vi "FL_Decode_RAW_to_DEC_2.vi"(0 "SB size (loc. var. only)":u8, 1 "IO ports config":bool[](array[boolean])=[TRUE, TRUE, FALSE, FALSE], 2 "Input string":string, 3 "Input timestamp":timestamp, 4 "IO inversion config.":u16, 5 "Error In":errorcluster) -> (6 "Output string leftover":string, 7 "DEC output cluster":T1, 8 "Error Out":errorcluster)   [LabVIEW 2018, in "Tracker.lvlib"]
uses:
  Tracker.lvlib
  Controls/CTL_Decoded_data_frame.ctl
panel:
  out "TTL ins":bool[](array[boolean])
  out "TTL outs":bool[](array[boolean])
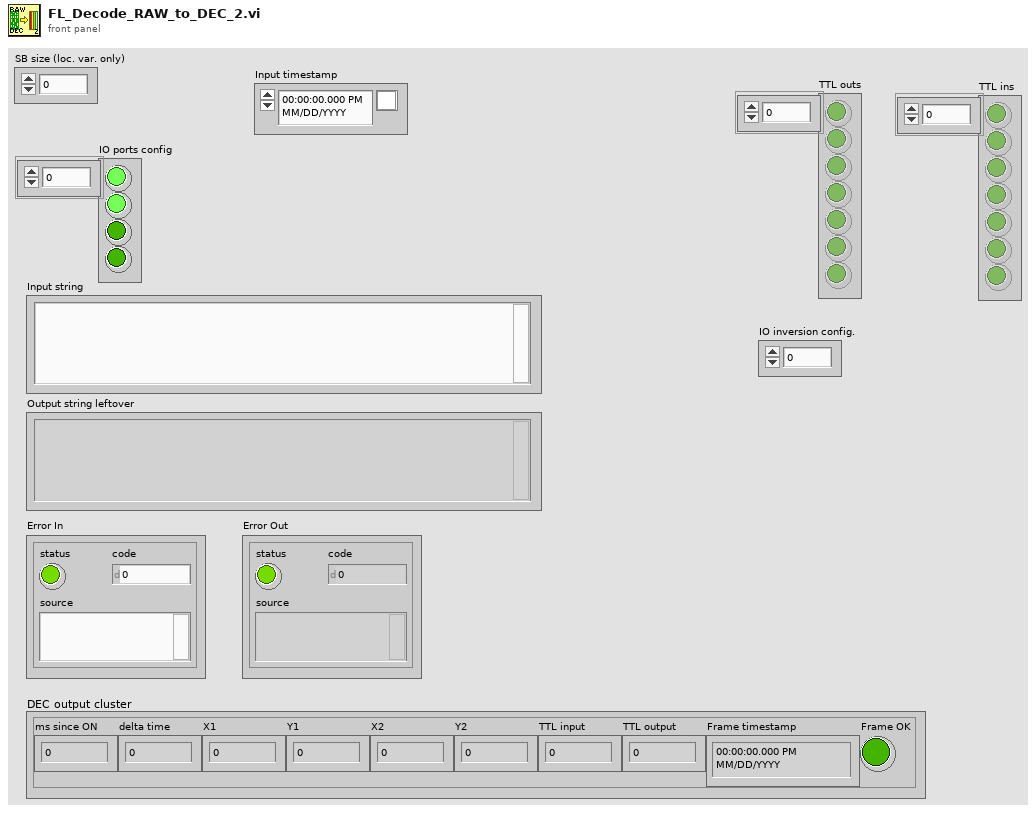
[diagram p1: front panel]
types:
  T1 = typedef "Tracker.lvlib/CTL_Decoded_data_frame.ctl" = cluster{"ms since ON":u32, "delta time":u32, "X1":sgl, "Y1":sgl, "X2":sgl, "Y2":sgl, "TTL input":i16, "TTL output":i16, "Frame timestamp":timestamp, "Frame OK":bool}
  T2 = cluster{"ms since ON":u32, "delta time":u32, "X1":sgl, "Y1":sgl, "X2":sgl, "Y2":sgl, "TTL inputs":u8, "TTL outputs":u8, "Frame timestamp":timestamp, "Frame OK":bool}
  T3 = cluster{"ms since ON":u32, "delta time":u32, "X1":sgl, "Y1":sgl, "X2":sgl, "Y2":sgl, "TTL IO status":u8, "Frame timestamp":timestamp, "Frame OK":bool}
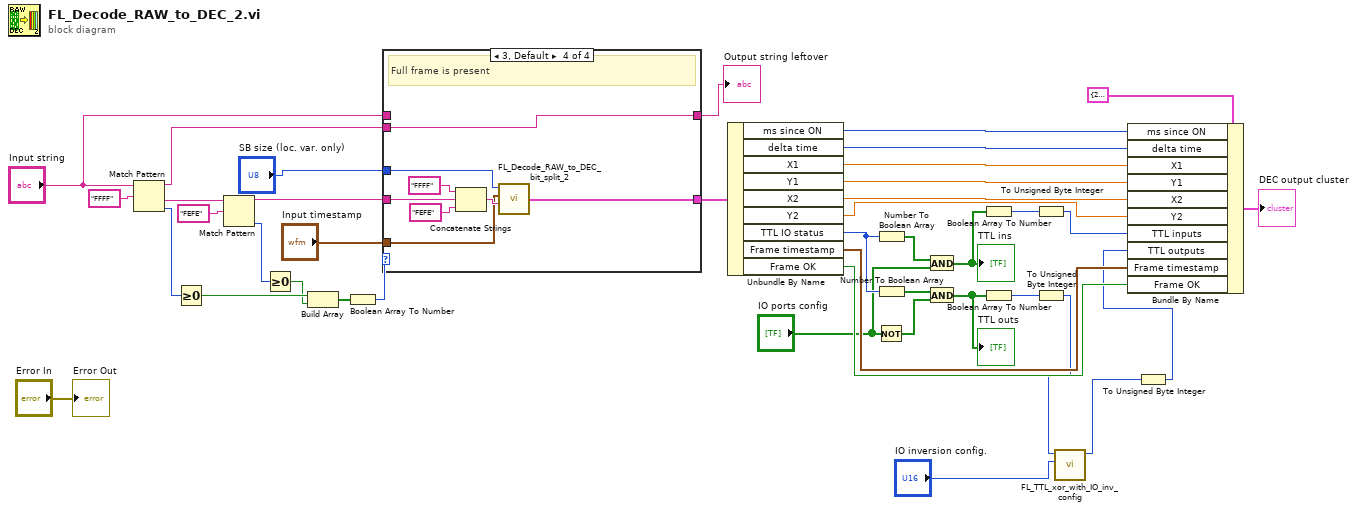
[diagram p0: block diagram]
diagram:
  n1 = Match Pattern(string="Input string", regular expression="FFFF") -> (before substring=w29:string, after substring=w30:string, offset past match=w34:i32)  [unwired: 1 in, 1 out]
  n2 = Greater Or Equal To 0?(x=w34) -> (x >= 0?=w39:bool)
  n3 = Match Pattern(string=w30, regular expression="FEFE") -> (before substring=w33:string, offset past match=w35:i32)  [unwired: 1 in, 2 out]
  n4 = Greater Or Equal To 0?(x=w35) -> (x >= 0?=w38:bool)
  n5 = Build Array(w39, w38) -> (w36:bool[])
  n6 = Boolean Array To Number(Boolean array=w36) -> (number=w37:u32)
  n7 = case shown="3, Default" w37 {
    tunnel: w33 -> [_ _ _ w51]
    tunnel: [_ _ _ w52] -> w26
    tunnel: "Input timestamp" -> [_ _ _ w46]
    tunnel: [w42 w43 w44 w47] -> w31
    tunnel: w29 -> [_ _ _ w47]
    tunnel: "Input string" -> [w42 w43 w44 _]
    tunnel: "SB size (loc. var. only)" -> [_ _ _ w45]
    frame 0 {
      # "Neither beginning, nor ending of frame is present"
    }
    frame 1 {
      # "Only frame beginning is present"
    }
    frame 2 {
      # "Only frame end is present"
    }
    frame 3, Default {
      # "Full frame is present"
      n8 = Concatenate Strings("FFFF" ("string"), w51, "FEFE" ("string")) -> (w50:string)
      n9 = call "FL_Decode_RAW_to_DEC_bit_split_2.vi"("Read buffer text to decode"=w50, "Input timestamp"=w46, "SB size (loc. var. only)"=w45) -> ("DEC output cluster"=w52:T3)  [unwired: 1 in]
    }
  }
  "Output string leftover" <- w31
  n10 = Unbundle By Name(w26) -> ("ms since ON"=w23:u32, "delta time"=w22:u32, "X1"=w21:sgl, "Y1"=w20:sgl, "X2"=w19:sgl, "Y2"=w18:sgl, "TTL IO status"=w14:u8, "Frame timestamp"=w17:timestamp, "Frame OK"=w16:bool)
  n11 = Not(x="IO ports config") -> (.not. x?=w11:bool[])
  n12 = Number To Boolean Array(number=w14) -> (Boolean array=w13:bool[])
  n13 = Number To Boolean Array(number=w14) -> (Boolean array=w15:bool[])
  n14 = And(x=w13, y="IO ports config") -> (x .and. y?=w8:bool[])
  "TTL ins" <- w8
  n15 = And(x=w15, y=w11) -> (x .and. y?=w10:bool[])
  "TTL outs" <- w10
  n16 = Boolean Array To Number(Boolean array=w8) -> (number=w7:u32)
  n17 = Boolean Array To Number(Boolean array=w10) -> (number=w9:u32)
  n18 = To Unsigned Byte Integer(number=w7) -> (unsigned 8bit integer=w6:u8)
  n19 = To Unsigned Byte Integer(number=w9) -> (unsigned 8bit integer=w4:u8)
  n20 = call "FL_TTL_xor_with_IO_inv_config.vi"("IO inversion config."="IO inversion config.", "TTL port(s) config to fire"=w4) -> ("ON config."=w3:u32)  [unwired: 8 in, 1 out]
  n21 = To Unsigned Byte Integer(number=w3) -> (unsigned 8bit integer=w2:u8)
  n22 = Bundle By Name(cluster=T2 {"ms since ON"=21424124, "delta time"=12, "X1"=-25.617287, "Y1"=-34.72222, "X2"=-30.650688, "Y2"=38.869858, "TTL inputs"=4, "TTL outputs"=0, "Frame timestamp"=timestamp(3611917532.9919057 s since 1904-01-01), "Frame OK"=TRUE} ("DEC output cluster"), "ms since ON"=w23, "delta time"=w22, "X1"=w21, "Y1"=w20, "X2"=w19, "Y2"=w18, "TTL inputs"=w6, "TTL outputs"=w2, "Frame timestamp"=w17, "Frame OK"=w16) -> (→"DEC output cluster":T2)
  "Error Out" <- "Error In"
